vi "Linearize Measure Evaluation.vi"(8 "step (m)":dbl=0.0001, 11 "Distance Array":dbl[](array[numeric])) -> (0 "Mean error (m)":dbl, 1 "RMS":dbl format="%0.2f", 2 "Max peak-peak error (m)":dbl, 3 "Regression curve":dbl[](array[numeric]))   [LabVIEW 2014]
uses:
  <vilib>/Analysis/5stat.llb/RMS (DBL).vi
  <vilib>/Analysis/baseanly.llb/Mean (DBL).vi
  <vilib>/Analysis/NI_AALBase.lvlib
  <vilib>/Analysis/NI_AALPro.lvlib
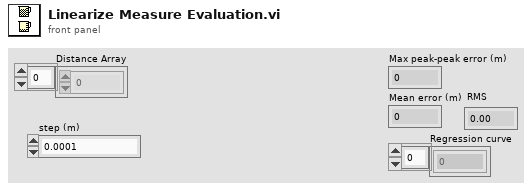
[diagram p1: front panel]
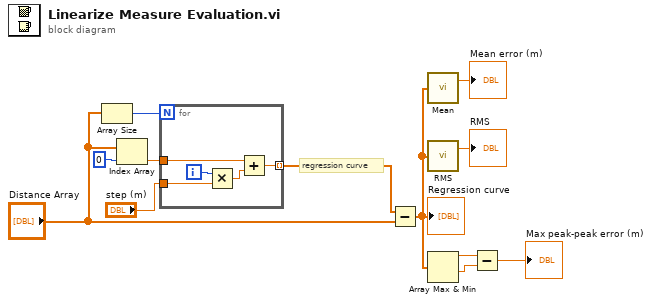
[diagram p0: block diagram]
diagram:
  # "regression curve"
  n1 = Array Size(array="Distance Array") -> (size(s)=w11:i32)
  n2 = Index Array(array="Distance Array", index=0) -> (element=w10:dbl)
  n3 = for {
    N: w11 -> [_]
    tunnel: w10 -> [w16]
    tunnel: [w14] -> w8 mode=indexing
    tunnel: "step (m)" -> [w13]
    i -> [w15]
    n4 = Multiply(x=w15, y=w13) -> (x*y=w17:dbl)
    n5 = Add(x=w16, y=w17) -> (x+y=w14:dbl)
  }
  n6 = Subtract(x=w8, y="Distance Array") -> (x-y=w2:dbl[])
  "Regression curve" <- w2
  n7 = call-poly <vilib>:"Mean.vi"("X"=w2) -> ("mean"=→"Mean error (m)":dbl)  [unwired: 1 out]
  n8 = call-poly <vilib>:"RMS.vi"("X"=w2) -> ("rms value"=→"RMS":dbl)  [unwired: 1 out]
  n9 = Array Max & Min(array=w2) -> (max value=w6:dbl, min value=w5:dbl)  [unwired: 2 out]
  n10 = Subtract(x=w6, y=w5) -> (x-y=→"Max peak-peak error (m)":dbl)
